vi "DAQNavi Write (Digital U8 1Chan 1Samp).vi"(7 "portBit":i32=-1, 8 "error in (no error)":errorcluster, 9 "timeout":dbl=10.0, 10 "data":u8, 11 "task in":i32) -> (0 "error out":errorcluster, 2 "number of samples written per channel":u32, 3 "task out":i32)   [LabVIEW 2020]
uses:
  DAQNavi_LV.dll
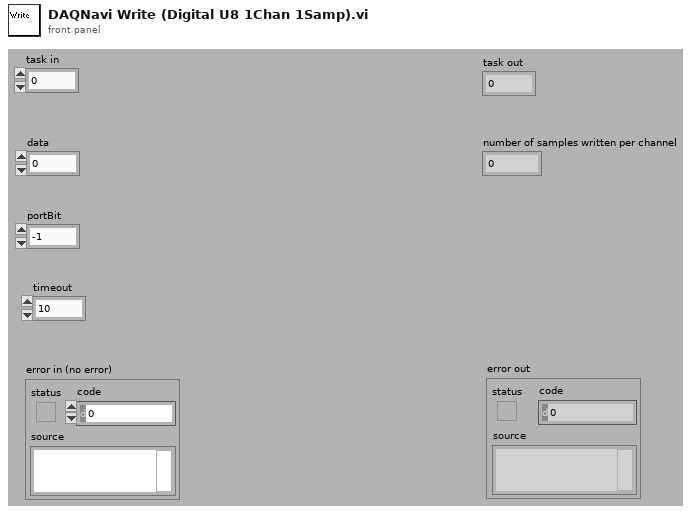
[diagram p1: front panel]
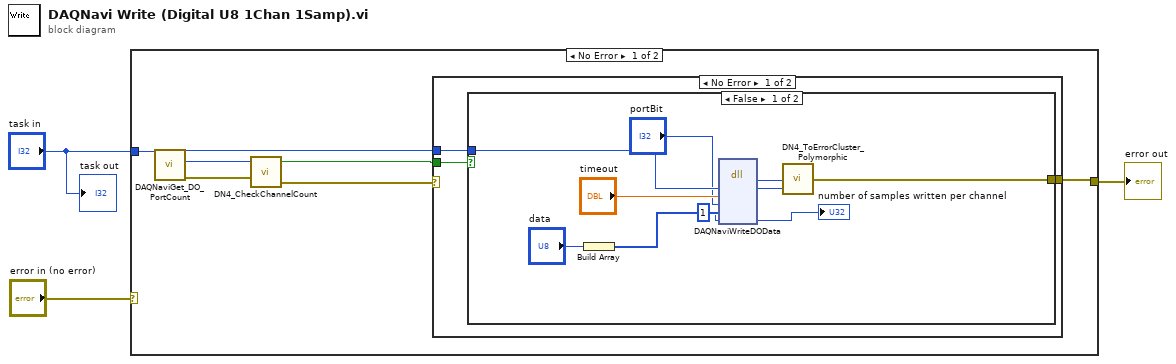
[diagram p0: block diagram]
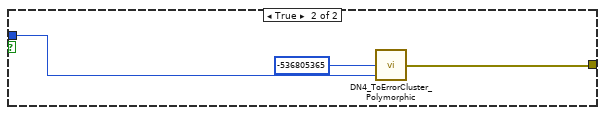
[diagram p2: hidden frame]
diagram:
  n1 = case shown="No Error" "error in (no error)" {
    selector: "error in (no error)" -> [_ w28]
    tunnel: [w9 w28] -> w2
    tunnel: "task in" -> [w10 _]
    frame No Error {
      n2 = call "DAQNaviGet_DO_PortCount.vi"("task in"=w10) -> ("error out"=w7:errorcluster, "port count"=w8:i32, "task out"=w4:i32)  [unwired: 1 in, 7 out]
      n3 = call "DN4_CheckChannelCount.vi"("error out"=w7, "channel count"=w8) -> ("error IO"=w5:errorcluster, "greater than 1?"=w6:bool)  [unwired: 2 out]
      n4 = case shown="No Error" w5 {
        selector: w5 -> [_ w27]
        tunnel: w6 -> [w13 _]
        tunnel: w4 -> [w12 _]
        tunnel: [w11 w27] -> w9
        frame No Error {
          n5 = case shown="False" w13 {
            tunnel: [w16 w25] -> w11
            tunnel: w12 -> [w23 w24]
            frame False {
              n6 = Build Array("data") -> (w20:u8[])
              n7 = dll-call lib="DAQNavi_LV.dll" fn="DAQNaviWriteDOData"("taskID"=w23, "timeout"="timeout", "portBit"="portBit", "portData"=w20, "samples"=u32 1) -> ("return type"=w17:i32, "taskID"=w15:i32, "samples"=→"number of samples written per channel":u32)  [unwired: 6 in, 2 out]
              n8 = call "DN4_ToErrorCluster_Polymorphic.vi"("task id"=w15, "error code"=w17) -> ("error out"=w16:errorcluster)  [unwired: 3 out]
            }
            frame True {
              n9 = call "DN4_ToErrorCluster_Polymorphic.vi"("task id"=w24, "error code"=-536805365 ("error code (0)")) -> ("error out"=w25:errorcluster)  [unwired: 3 out]
            }
          }
        }
        frame Error {
        }
      }
    }
    frame Error {
    }
  }
  "error out" <- w2
  "task out" <- "task in"
